vi "InstrParam.vi"(4 "queue out":refnum<queue>, 6 "user event out":refnum<user-event>, 8 "error in (no error)":errorcluster caption="entrée d'erreur (pas d'erreur)", 10 "InstrParam":string, 11 "Taiko en entrée":refnum<class "TaikoLaser.lvclass"> caption="DNL_LabVIEW Object in") -> (0 "error out":errorcluster caption="sortie d'erreur", 3 "Taiko en sortie":refnum<class "TaikoLaser.lvclass"> caption="DNL_LabVIEW Object out")   [LabVIEW 2019, in "TaikoLaser.lvclass"]
uses:
  TaikoLaser.lvclass
  C:/Programmes Labview/LabscanV1A/DevicesClass/BaseDevice/BaseDevice.lvclass
  BaseDevice/ClassQueueMess.ctl
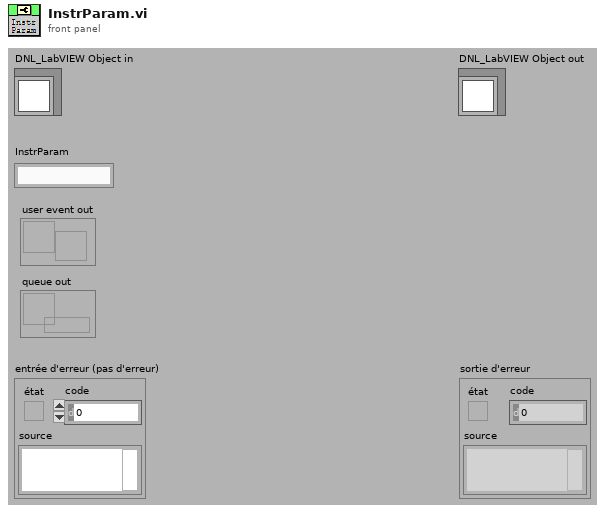
[diagram p1: front panel]
types:
  T1 = typedef "ClassQueueMess.ctl" = u16
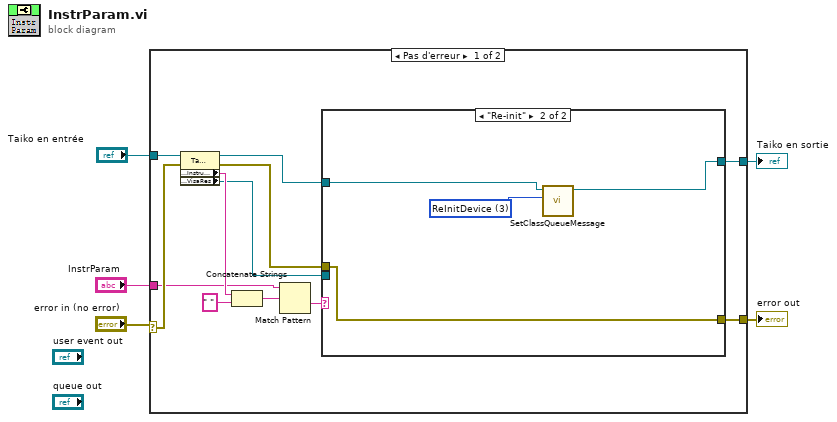
[diagram p0: block diagram]
diagram:
  n1 = case shown="Pas d'erreur" "error in (no error)" {
    selector: "error in (no error)" -> [w16 w24]
    tunnel: "Taiko en entrée" -> [w17 w25]
    tunnel: [w12 w25] -> w3
    tunnel: [w9 w24] -> w2
    tunnel: "InstrParam" -> [w6 _]
    frame No Error {
      n2 = property class="TaikoLaser.lvclass"(reference=w17, error in=w16) -> (reference out=w11:refnum<class "TaikoLaser.lvclass">, error out=w10:errorcluster, "Accessor:InstrumentName"=w14:string, "Accessor:VisaRes"=w8:refnum<visa-resource-name>)
      n3 = Concatenate Strings(w14, " " ("chaîne")) -> (w7:string)
      n4 = Match Pattern(string=w6, regular expression=w7) -> (after substring=w13:string)  [unwired: 1 in, 3 out]
      n5 = case shown="\"Re-init\"" w13 {
        tunnel: [w19 w21] -> w12
        tunnel: w11 -> [w19 w22]
        tunnel: w10 -> [w18 w23]
        tunnel: [w18 w23] -> w9
        tunnel: w8 -> [_ _]
        frame Default {
        }
        frame "Re-init" {
          w20 = T1 3 items=["UpdateClassData", "UpdateMainClass", "UpdateDataBind", "ReInitDevice"] ("Menu déroulant")
          n6 = call-dynamic "SetClassQueueMessage.vi"("Menu déroulant"=w20, "DefaultDev.lvclass"=w22) -> ("DefaultDev.lvclass Out"=w21:refnum<class "TaikoLaser.lvclass">)  [unwired: 8 in, 1 out]
        }
      }
    }
    frame Error {
    }
  }
  "error out" <- w2
  "Taiko en sortie" <- w3
